vi "velRaw_to_useful.vi"(8 "timeInterval (ms)":dbl=100.0, 9 "ticksPerRot":dbl=4096.0, 11 "rawUnits":dbl) -> (0 "FPS_vel":dbl, 2 "RPS_vel":dbl, 3 "RPM_vel":dbl)   [LabVIEW 2017]
panel:
  in  "wheelDiameter (in)":dbl
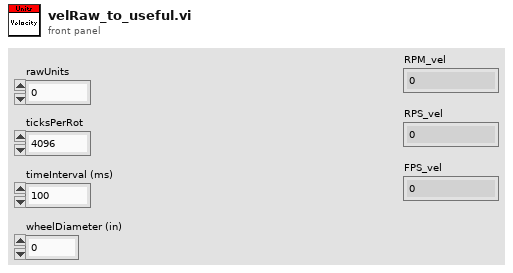
[diagram p1: front panel]
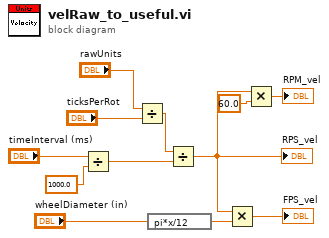
[diagram p0: block diagram]
diagram:
  n1 = Divide(x="timeInterval (ms)", y=1000.0) -> (x/y=w7:dbl)
  n2 = Divide(x="rawUnits", y="ticksPerRot") -> (x/y=w8:dbl)
  n3 = expression code="pi*x/12"("wheelDiameter (in)") -> (w2:dbl)
  n4 = Divide(x=w8, y=w7) -> (x/y=w3:dbl)
  "RPS_vel" <- w3
  n5 = Multiply(x=w3, y=w2) -> (x*y=→"FPS_vel":dbl)
  n6 = Multiply(x=w3, y=60.0) -> (x*y=→"RPM_vel":dbl)
